vi "Append Terminating Character for Write Command.vi"(1 "Command in":string) -> (0 "Command with Terminating character out":string)   [LabVIEW 2018]
doc: "Appends the terminating character to the write command on the universal electric actuator.\n\n\n(Nimble Focus Consulting 2019)"
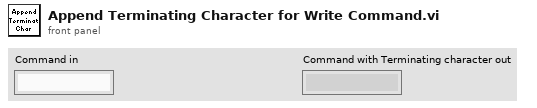
[diagram p1: front panel]
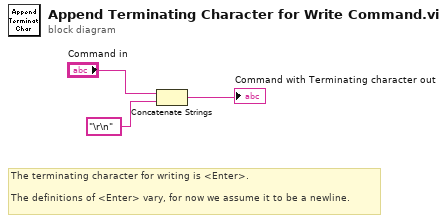
[diagram p0: block diagram]
diagram:
  # "The terminating character for writing is <Enter>.\n\nThe definitions of <Enter> vary, for now we assume it to be a newline."
  n1 = Concatenate Strings("Command in", "\r\n") -> (→"Command with Terminating character out":string)
